vi "HOST_GLOBAL.vi"() -> ()   [LabVIEW 2023]
panel:
  out "Connected":bool
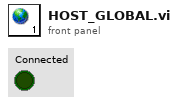
[diagram p1: front panel]
diagram:
